vi "Database_Ops.vi"(7 "Record data":string[](array[string])=["Vaddio 6940-001", "1.1", "997-6940-001", "1A", "2013-07-23", "Joe", "WO12345", "123456789", "None", "5:31", "Pass", "12.3vdc", "12mA", "4 sec", "245 ohm", "121vac", "2.1 vPP", "", "", "", "", "", "", "", "", "", "", "", "", "", "", "", "", "", "", "", "", "", "", "", "", "", "", "", "", "", "", "", "", "", "", "", "", "", "", "", "", "", "", "", "", "", "12:01:00"], 8 "Error in (no error)":errorcluster, 9 "SQL Query":string="Select * from BTWtestREC where Date >= '2013-07-24'", 10 "ConnectionString":string="Provider=SQLNCLI11.1;Integrated Security=SSPI;Persist Security Info=False;User ID=\"\";Initial Catalog=BTW_TEST;Data Source=TEST-LAPTOP\\SQLEXPRESS;Initial File Name=\"\";Server SPN=\"\"", 11 "Operation":T1(ring)=enum."Select") -> (0 "Error out":errorcluster, 1 "Rec Count":string="0", 2 "Column Names":string[](array[string])=["UniqueID", "Program", "ProgramRev", "PartNumber", "PartRev", "Date", "Operator", "WorkOrder", "SerialNumber", "Address", "ExecuteTime", "UutResult", "Results", "Result1", "Result2", "Result3", "Result4", "Result5", "Result6", "Result7", "Result8", "Result9", "Result10", "Result11", "Result12", "Result13", "Result14", "Result15", "Result16", "Result17", "Result18", "Result19", "Result20", "Result21", "Result22", "Result23", "Result24", "Result25", "Result26", "Result27", "Result28", "Result29", "Result30", "Result31", "Result32", "Result33", "Result34", "Result35", "Result36", "Result37", "Result38", "Result39", "Result40", "Result41", "Result42", "Result43", "Result44", "Result45", "Result46", "Result47", "Result48", "Result49", "Result50", "Time"], 3 "RecordSet":string[][](array[string]))   [LabVIEW 2013]
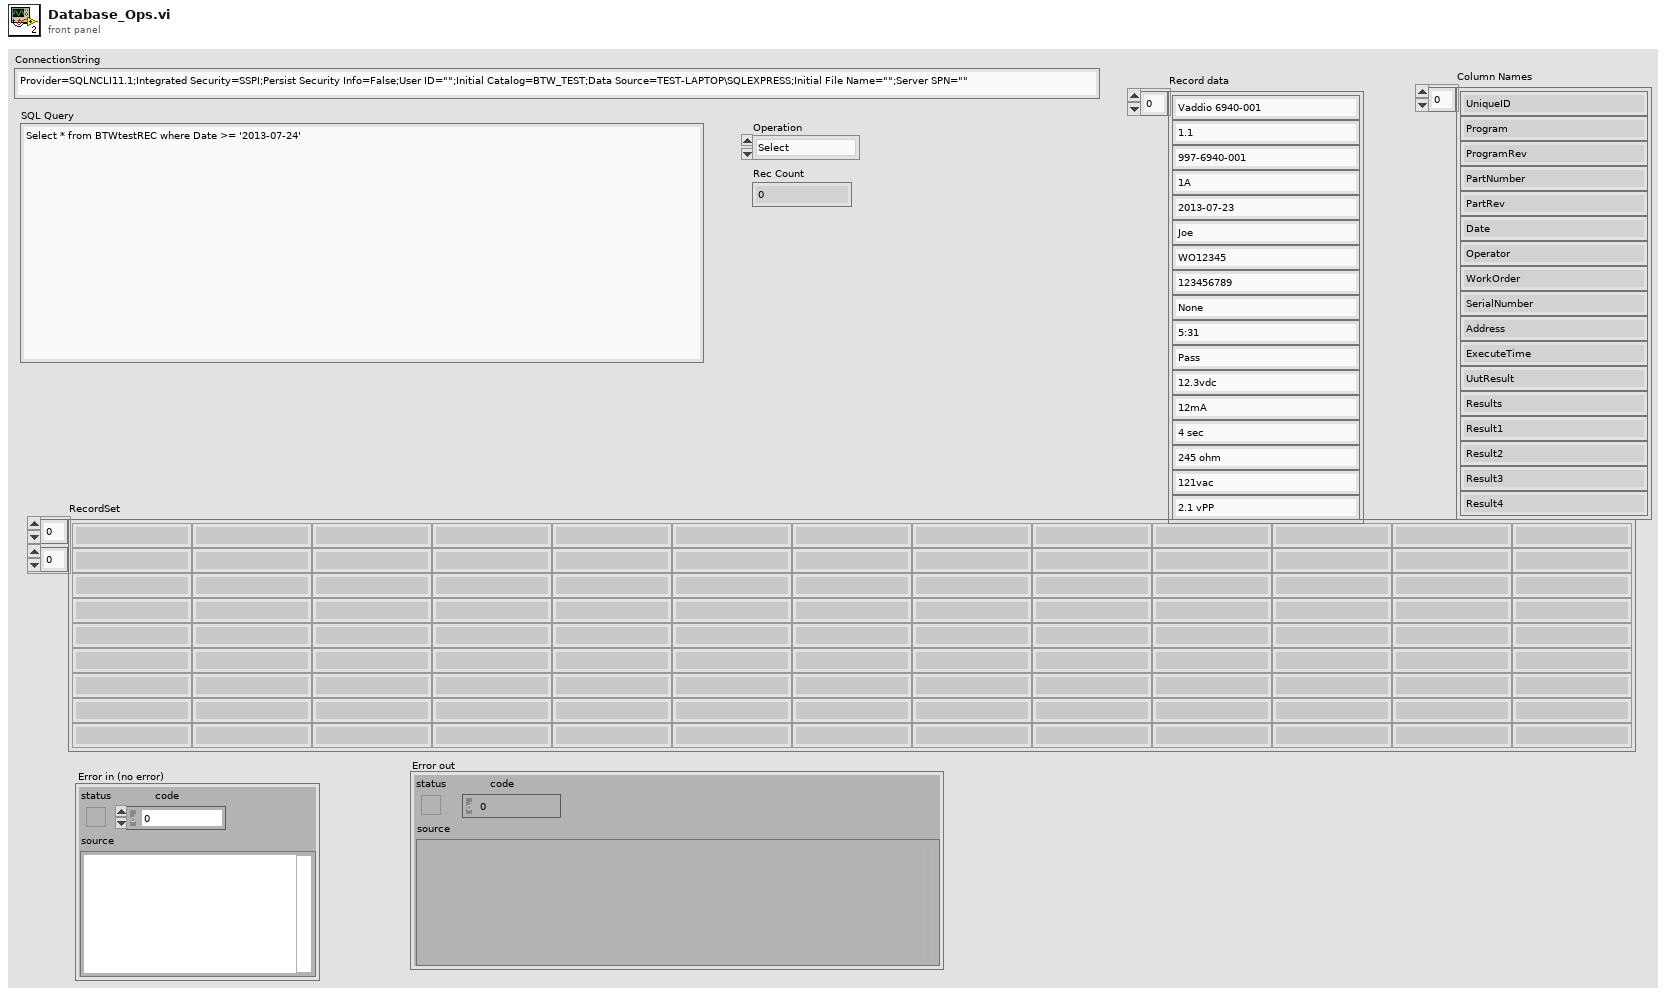
[diagram p1: front panel]
types:
  T1 = enum16{"Query", "Insert", "Select", "Dump Recs", "Get Rec Count", "Get Col Names"}
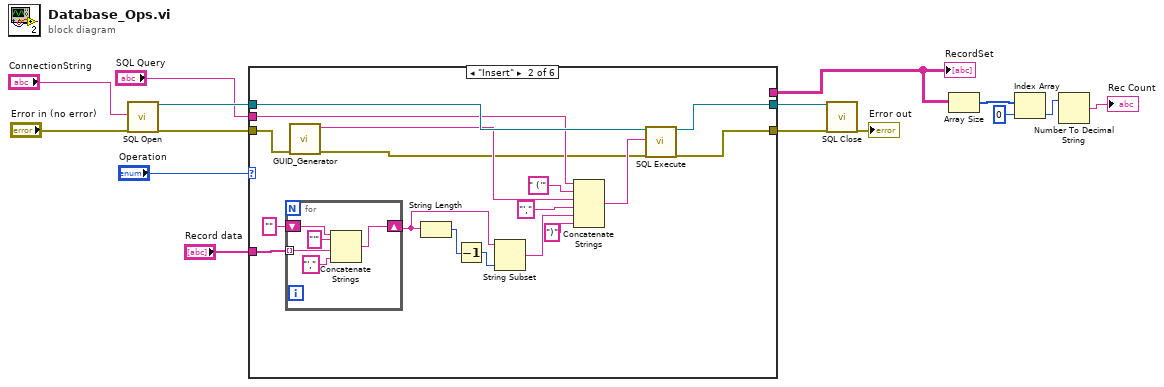
[diagram p0: block diagram]
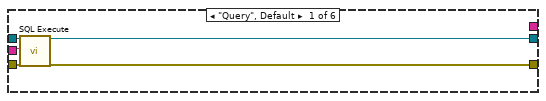
[diagram p2: hidden frame]
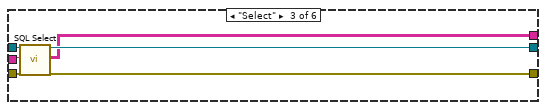
[diagram p3: hidden frame]
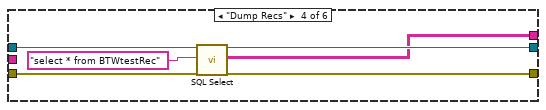
[diagram p4: hidden frame]
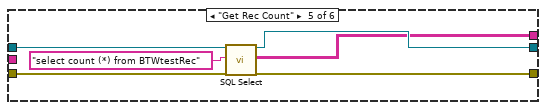
[diagram p5: hidden frame]
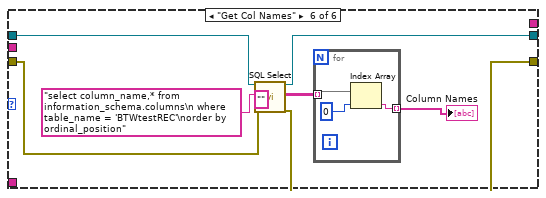
[diagram p6: hidden frame]
diagram:
  n1 = call "SQL Open.vi"("ConnectionString In"="ConnectionString", "Error in (no error)"="Error in (no error)") -> ("Connection Out"=w11:refnum<k7>, "Error out"=w10:errorcluster)  [unwired: 16 in]
  n2 = case shown="\"Insert\"" "Operation" {
    tunnel: [w17 w37 w44 w51 w56 w62] -> w13
    tunnel: [w16 w36 w45 w52 w57 w61] -> w12
    tunnel: w11 -> [w19 w35 w46 w54 w60 w66]
    tunnel: w10 -> [w18 w34 w48 w53 w59 w65]
    tunnel: "SQL Query" -> [w20 w28 w47 _ _ _]
    tunnel: [_ _ w43 w49 w55 _] -> w5
    tunnel: "Record data" -> [_ w33 _ _ _ _]
    frame "Query", Default {
      n3 = call "SQL Execute.vi"("Connection In"=w19, "SQL Query"=w20, "Error in (no error)"=w18) -> ("Connection Out"=w16:refnum<k7>, "Error out"=w17:errorcluster)  [unwired: 15 in]
    }
    frame "Insert" {
      n4 = for {
        tunnel: w33 -> [w42] mode=indexing
        shift-right: [w40] -> w22
        shift-left: "" -> [w39]
        n5 = Concatenate Strings(w39, "'" ("string"), w42, "'," ("string")) -> (w40:string)
      }
      n6 = call "GUID_Generator.vi"("error in (no error)"=w34) -> ("error out"=w26:errorcluster, "GUID String"=w32:string)  [unwired: 9 in]
      n7 = String Length(string=w22) -> (length=w24:i32)
      n8 = Decrement(x=w24) -> (x-1=w23:i32)
      n9 = String Subset(string=w22, length (rest)=w23) -> (substring=w21:string)  [unwired: 1 in]
      n10 = Concatenate Strings(w28, " ('" ("string"), w32, "'," ("string"), w21, ")") -> (w27:string)
      n11 = call "SQL Execute.vi"("Connection In"=w35, "SQL Query"=w27, "Error in (no error)"=w26) -> ("Connection Out"=w36:refnum<k7>, "Error out"=w37:errorcluster)  [unwired: 15 in]
    }
    frame "Select" {
      n12 = call "SQL Select.vi"("Connection In"=w46, "SQL Query"=w47, "Error in (no error)"=w48) -> ("Connection Out"=w45:refnum<k7>, "Data"=w43:string[][], "Error out"=w44:errorcluster)  [unwired: 14 in]
    }
    frame "Dump Recs" {
      n13 = call "SQL Select.vi"("Connection In"=w54, "SQL Query"="select * from BTWtestRec", "Error in (no error)"=w53) -> ("Connection Out"=w52:refnum<k7>, "Data"=w49:string[][], "Error out"=w51:errorcluster)  [unwired: 14 in]
    }
    frame "Get Rec Count" {
      n14 = call "SQL Select.vi"("Connection In"=w60, "SQL Query"="select count (*) from BTWtestRec", "Error in (no error)"=w59) -> ("Connection Out"=w57:refnum<k7>, "Data"=w55:string[][], "Error out"=w56:errorcluster)  [unwired: 14 in]
    }
    frame "Get Col Names" {
      (unwired) "" ("SQL Query")
      n15 = call "SQL Select.vi"("Connection In"=w66, "SQL Query"="select column_name,* from information_schema.columns\n where table_name = 'BTWtestREC'\norder by ordinal_position", "Error in (no error)"=w65) -> ("Connection Out"=w61:refnum<k7>, "Data"=w64:string[][], "Error out"=w62:errorcluster)  [unwired: 14 in]
      n16 = for {
        tunnel: w64 -> [w70] mode=indexing
        tunnel: [w69] -> w63 mode=indexing
        n17 = Index Array(array=w70, index=0 ("index (col)")) -> (element=w69:string)
      }
      "Column Names" <- w63
    }
  }
  "RecordSet" <- w5
  n18 = call "SQL Close.vi"("Connection In"=w12, "Error in (no error)"=w13) -> ("Error out"=→"Error out":errorcluster)  [unwired: 17 in]
  n19 = Array Size(array=w5) -> (size(s)=w4:i32[])
  n20 = Index Array(array=w4, index=0) -> (element=w3:i32)
  n21 = Number To Decimal String(number=w3) -> (decimal integer string=→"Rec Count":string)  [unwired: 1 in]
